vi "EyeTracking.vi"() -> ()   [LabVIEW 2010]
uses:
  <vilib>/vision/driver/IMAQdx.llb/IMAQdx Camera Control Mode.ctl
  <vilib>/vision/driver/NI_Vision_Acquisition_Software.lvlib
  Program Files/National Instruments/LabVIEW 2010/resource/objmgr/imaqdx.rc
  <vilib>/vision/driver/IMAQdx.llb/IMAQdx Acquisition Mode.ctl
  <vilib>/vision/NI_Vision_Development_Module.lvlib
  <vilib>/Utility/Variable/NI_VariableUtilities.lvlib
  <vilib>/DAQmx/write.llb/DAQmx Write (Analog 1D DBL NChan 1Samp).vi
  <vilib>/userDefined/High Color/IMAQdx.ctl
panel:
  out "IMAQ":bool
  out "acquired FPS":dbl
  out "processed FPS":dbl
  in  "Range":cluster{"Lower value":sgl, "Upper value":sgl}={"Lower value"=0.0, "Upper value"=29.0}
  in  "update FPS":u32=30
  out "Eye Trace":dbl[][](graph)
  in  "Pupil Color":sgl=150.0
  out "Centroid":cluster{"X Centroid":sgl, "Y Centroid":sgl} {"Y Centroid" format="%.2f"; "X Centroid" format="%.2f"}
  in  "Min Size":dbl=300.0
  in  "Max Size":dbl=25000.0
  in  "Despeckle":bool
  in  "desired FPS":dbl=200.0
  in  "AO Task":refnum<k21>="OpticalTrackerOut"
  in  "Track":bool
  out "Image":T1(plugin-control)
  in  "Session In":T2="cam0"
  in  "stop":bool
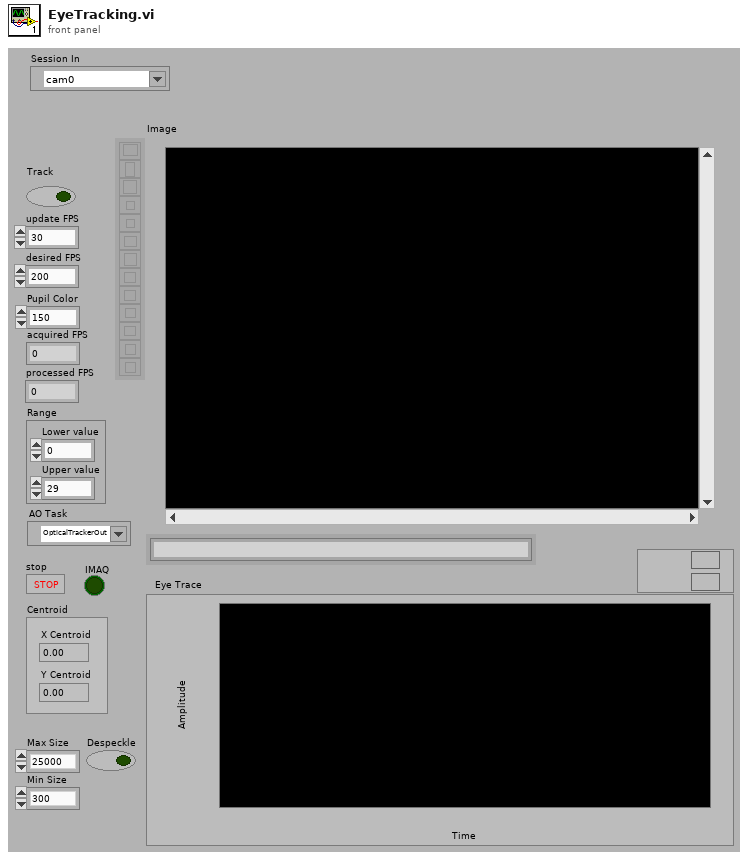
[diagram p1: front panel]
types:
  T1 = typedef "IMAQ Image.ctl" = refnum<image>
  T2 = typedef "IMAQdx.ctl" = refnum<k21>
  T3 = typedef "Image Type" = u32
  T4 = enum16{"Track", "Init Tracking", "Preview", "Init Preview"}
  T5 = cluster{"Type":u32, "Version":u32, "Flags":u32, "SerialNumberHigh":u32, "SerialNumberLow":u32, "BusType":u32, "InterfaceName":string, "VendorName":string, "ModelName":string, "CameraFileName":string, "CameraAttributeURL":string}[]
  T6 = typedef "NI_Vision_Acquisition_Software.lvlib/IMAQdx Camera Control Mode.ctl" = enum32{"Controller", "Listener"}
  T7 = typedef "NI_Vision_Acquisition_Software.lvlib/IMAQdx Acquisition Mode.ctl" = enum32{"One Shot", "Continuous"}
  T8 = cluster{"Global Rectangle":i32[], "Contours":cluster{"Contour Type":u32, "ROI Type":u32, "Points":i32[]}[]}
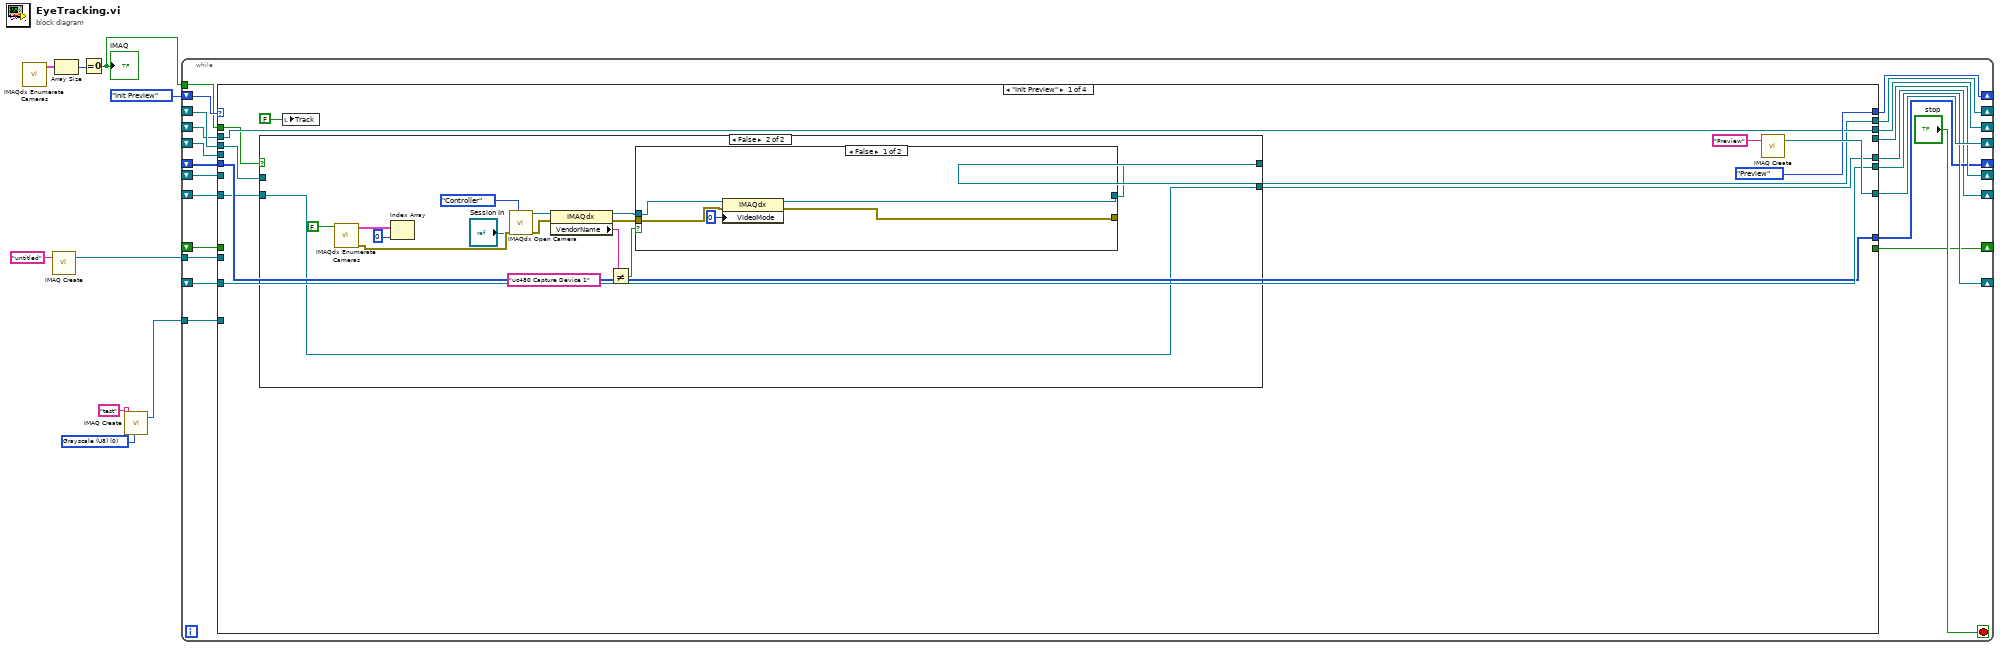
[diagram p0: block diagram]
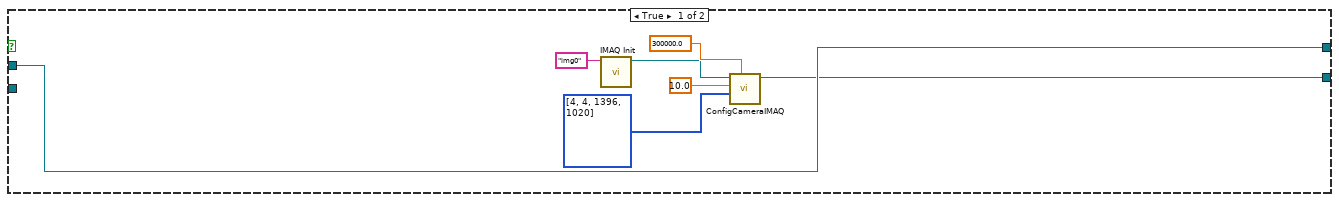
[diagram p2: hidden frame]
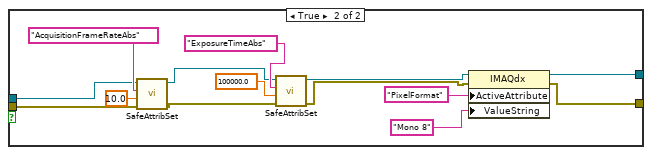
[diagram p3: hidden frame]
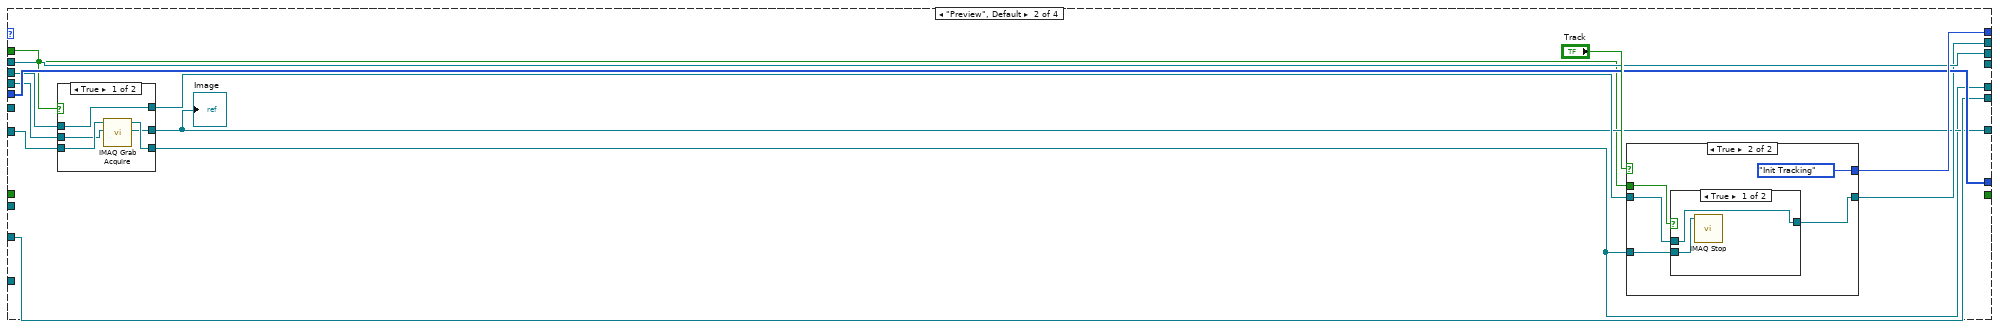
[diagram p4: hidden frame]
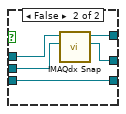
[diagram p5: hidden frame]
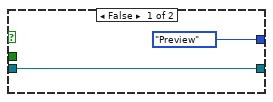
[diagram p6: hidden frame]
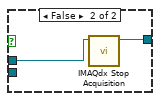
[diagram p7: hidden frame]
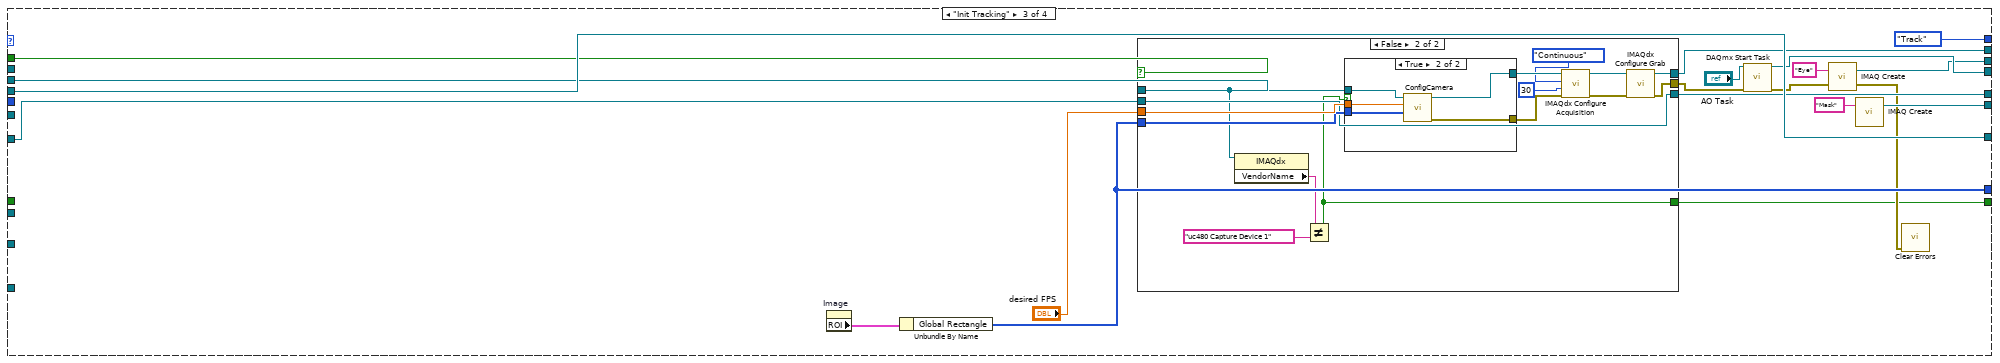
[diagram p8: hidden frame]
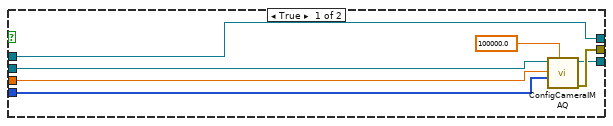
[diagram p9: hidden frame]
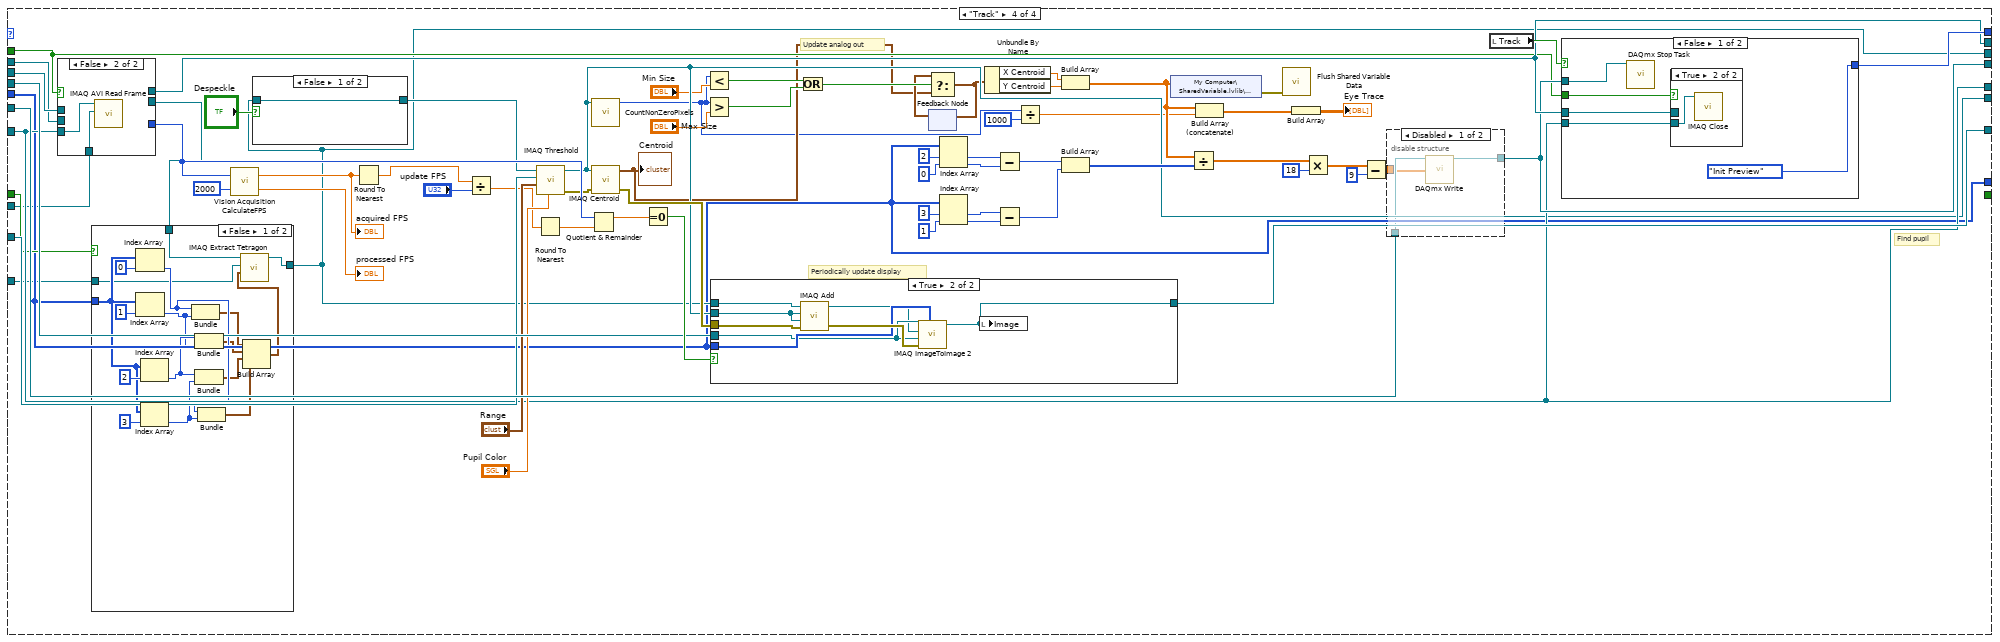
[diagram p11: hidden frame]
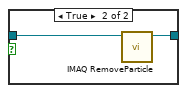
[diagram p14: hidden frame]
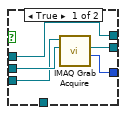
[diagram p15: hidden frame]
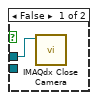
[diagram p17: hidden frame]
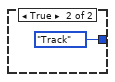
[diagram p18: hidden frame]
diagram:
  w5 = T3 0 items=["Grayscale (U8)", "Grayscale (I16)", "Grayscale (SGL)", "Complex (CSG)", "RGB (U32)", "HSL (U32)", "RGB (U64)", "Grayscale (U16)"] ("Image Type")
  n1 = call <vilib>:"IMAQdx Enumerate Cameras.vi"() -> ("Camera Information Array"=w8:T5)  [unwired: 2 in, 9 out]
  n2 = call "IMAQ Create"("Image Name"="untitled") -> ("New Image"=w1:T1)  [unwired: 4 in, 1 out]
  n3 = Array Size(array=w8) -> (size(s)=w7:i32)
  n4 = Equal To 0?(x=w7) -> (x = 0?=w6:bool)
  "IMAQ" <- w6
  n5 = call "IMAQ Create"("Image Name"="test", "Image Type"=w5) -> ("New Image"=w3:T1)  [unwired: 3 in, 1 out]
  n6 = while {
    shift-right: [w29] -> _
    shift-left: _ -> [w28]
    shift-right: [w27] -> _
    shift-left: _ -> [w26]
    shift-right: [w25] -> _
    shift-left: T4."Init Preview" -> [w30]
    shift-right: [w24] -> _
    shift-left: _ -> [w23]
    shift-right: [w22] -> _
    shift-left: _ -> [w21]
    shift-right: [w20] -> _
    shift-left: _ -> [w19]
    shift-right: [w18] -> _
    shift-left: _ -> [w17]
    tunnel: w6 -> [w16]
    shift-right: [w15] -> _
    shift-left: _ -> [w14]
    shift-right: [w13] -> _
    shift-left: _ -> [w12]
    tunnel: w3 -> [w11]
    tunnel: w1 -> [w10]
    stop <- "stop" stop-if-true
    n7 = case shown="\"Init Preview\"" w30 {
      tunnel: [w36 w88 w134 w229] -> w29
      tunnel: w28 -> [w34 w91 w123 w230]
      tunnel: [w42 w87 w136 w219] -> w27
      tunnel: w26 -> [_ w90 w136 w221]
      tunnel: [T4."Preview" w95 T4."Track" w232] -> w25
      tunnel: [_ _ w131 w225] -> w24
      tunnel: w23 -> [_ _ _ w228]
      tunnel: [w40 w94 w127 w169] -> w22
      tunnel: w21 -> [w40 w94 _ w220]
      tunnel: [w39 w92 w125 w188] -> w20
      tunnel: w19 -> [w39 w92 _ w202]
      tunnel: [w38 w93 w124 w168] -> w18
      tunnel: w17 -> [w38 w93 _ w168]
      tunnel: w16 -> [w35 w85 w122 w193]
      tunnel: [w33 w84 w120 w192] -> w15
      tunnel: w14 -> [w32 w86 w121 w192]
      tunnel: [_ _ w118 _] -> w13
      tunnel: w12 -> [_ _ _ w171]
      tunnel: w11 -> [_ _ _ w167]
      tunnel: w10 -> [_ _ _ w166]
      frame "Init Preview" {
        n8 = case shown="False" w35 {
          tunnel: [w50 w51] -> w36
          tunnel: w34 -> [w50 _]
          tunnel: [w46 w59] -> w33
          tunnel: w32 -> [_ w59]
          frame True {
            n9 = call <vilib>:"IMAQ Init.vi"("Interface Name"="img0") -> ("IMAQ Session Out"=w44:refnum<k11>)  [unwired: 1 in, 9 out]
            n10 = call "ConfigCameraIMAQ.vi"("desired exposure"=300000.0, "ROI"=i32[] [4, 4, 1396, 1020], "desired FPS"=10.0, "IMAQ Session In"=w44) -> ("IMAQ Session Out"=w46:refnum<k11>)  [unwired: 1 in, 6 out]
          }
          frame False {
            n11 = call <vilib>:"IMAQdx Enumerate Cameras.vi"("Connected Only? (Yes)"=FALSE) -> ("error out"=w61:errorcluster, "Camera Information Array"=w63:T5)  [unwired: 1 in, 8 out]
            n12 = Index Array(array=w63, index=0) -> ()  [unwired: 1 out]
            n13 = call <vilib>:"IMAQdx Open Camera.vi"("Camera Control Mode"=IMAQdx_Camera_Control_Mode."Controller", "error in"=w61, "Session In"="Session In") -> ("error out"=w56:errorcluster, "Session Out"=w57:T2)  [unwired: 7 out]
            n14 = property class="IMAQdx"(reference=w57, error in=w56) -> (error out=w55:errorcluster, "VendorName"=w54:string)  [unwired: 1 out]
            n15 = Not Equal?(x=w54, y="uc480 Capture Device 1") -> (x != y?=w53:bool)
            n16 = case shown="False" w53 {
              tunnel: [w67 w70] -> w51
              tunnel: [w66 w71] -> _
              tunnel: w57 -> [w69 w81]
              tunnel: w55 -> [w65 w80]
              frame False {
                n17 = property class="IMAQdx"(reference=w69, error in=w65, "VideoMode"=u32 0) -> (reference out=w67:T2, error out=w66:errorcluster)
              }
              frame True {
                n18 = call "SafeAttribSet.vi"("error in (no error)"=w80, "value"=10.0, "ActiveAttribute"="AcquisitionFrameRateAbs", "IMAQdx Session In"=w81) -> ("error out"=w76:errorcluster, "IMAQdx Session Out"=w77:T2)  [unwired: 6 out]
                n19 = call "SafeAttribSet.vi"("error in (no error)"=w76, "value"=100000.0, "ActiveAttribute"="ExposureTimeAbs", "IMAQdx Session In"=w77) -> ("error out"=w73:errorcluster, "IMAQdx Session Out"=w74:T2)  [unwired: 6 out]
                n20 = property class="IMAQdx"(reference=w74, error in=w73, "ActiveAttribute"="PixelFormat", "ValueString"="Mono 8") -> (reference out=w70:T2, error out=w71:errorcluster)
              }
            }
          }
        }
        n21 = local write "Track"(FALSE ("Track")) -> ()
        n22 = call "IMAQ Create"("Image Name"="Preview") -> ("New Image"=w42:T1)  [unwired: 3 in, 2 out]
      }
      frame "Preview", Default {
        n23 = case shown="True" w85 {
          tunnel: w91 -> [w101 w106]
          tunnel: [w98 w105] -> w87
          tunnel: w90 -> [w97 w104]
          tunnel: [w101 w103] -> w89
          tunnel: w86 -> [w100 w102]
          tunnel: [w99 w102] -> w84
          frame True {
            n24 = call <vilib>:"IMAQ Grab Acquire.vi"("Image In"=w97, "IMAQ Session In"=w100) -> ("Image Out"=w98:T1, "IMAQ Session Out"=w99:refnum<k11>)  [unwired: 3 in, 5 out]
          }
          frame False {
            n25 = call <vilib>:"IMAQdx Snap.vi"("Image In"=w104, "Session In"=w106) -> ("Image Out"=w105:T1, "Session Out"=w103:T2)  [unwired: 1 in, 7 out]
          }
        }
        "Image" <- w87
        n26 = case shown="True" "Track" {
          tunnel: [T4."Preview" T4."Init Tracking"] -> w95
          tunnel: w89 -> [w107 w112]
          tunnel: [w107 w111] -> w88
          tunnel: w85 -> [_ w110]
          tunnel: w84 -> [_ w109]
          frame False {
          }
          frame True {
            n27 = case shown="True" w110 {
              tunnel: w112 -> [w115 w117]
              tunnel: [w115 w116] -> w111
              tunnel: w109 -> [w114 _]
              frame True {
                n28 = call <vilib>:"IMAQ Stop.vi"("IMAQ Session In"=w114) -> ()  [unwired: 1 in, 10 out]
              }
              frame False {
                n29 = call <vilib>:"IMAQdx Stop Acquisition.vi"("Session In"=w117) -> ("Session Out"=w116:T2)  [unwired: 1 in, 9 out]
              }
            }
          }
        }
      }
      frame "Init Tracking" {
        n30 = property on="Image" class="ImageControl"() -> ("ROI"=w137:T8)  [unwired: 2 in, 2 out]
        n31 = Unbundle By Name(w137) -> ("Global Rectangle"=w124:i32[])
        n32 = case shown="False" w122 {
          tunnel: [w139 w159] -> w134
          tunnel: "desired FPS" -> [w143 w158]
          tunnel: [w141 w157] -> w130
          tunnel: w124 -> [w142 w156]
          tunnel: w123 -> [w139 w148]
          tunnel: w121 -> [w144 w151]
          tunnel: [w140 w151] -> w120
          tunnel: [_ w145] -> w118
          frame True {
            n33 = call "ConfigCameraIMAQ.vi"("desired exposure"=100000.0, "ROI"=w142, "desired FPS"=w143, "IMAQ Session In"=w144) -> ("error out"=w141:errorcluster, "IMAQ Session Out"=w140:refnum<k11>)  [unwired: 1 in, 5 out]
          }
          frame False {
            n34 = property class="IMAQdx"(reference=w148) -> ("VendorName"=w150:string)  [unwired: 1 in, 2 out]
            n35 = Not Equal?(x=w150, y="uc480 Capture Device 1") -> (x != y?=w145:bool)
            n36 = case shown="True" w145 {
              tunnel: w158 -> [_ w165]
              tunnel: w156 -> [_ w164]
              tunnel: [w160 w163] -> w155
              tunnel: [_ w162] -> w153
              tunnel: w148 -> [w160 w161]
              frame False {
              }
              frame True {
                n37 = call "ConfigCamera.vi"("ROI"=w164, "desired FPS"=w165, "Session In"=w161) -> ("error out"=w162:errorcluster, "IMAQdx Session Out"=w163:T2)  [unwired: 1 in, 6 out]
              }
            }
            n38 = call <vilib>:"IMAQdx Configure Acquisition.vi"("error in"=w153, "Number of Buffers"=u32 30, "Continuous?"=IMAQdx_Acquisition_Mode."Continuous", "Session In"=w155) -> ("error out"=w152:errorcluster, "Session Out"=w154:T2)  [unwired: 6 out]
            n39 = call <vilib>:"IMAQdx Configure Grab.vi"("error in"=w152, "Session In"=w154) -> ("error out"=w157:errorcluster, "Session Out"=w159:T2)  [unwired: 8 out]
          }
        }
        n40 = call <vilib>:"DAQmx Start Task.vi"("task/channels in"="AO Task", "error in"=w130) -> ("task out"=w131:refnum<k21>, "error out"=w128:errorcluster)  [unwired: 12 out]
        n41 = call "IMAQ Create"("Image Name"="Eye", "error in (no error)"=w128) -> ("New Image"=w127:T1, "error out"=w119:errorcluster)  [unwired: 2 in, 1 out]
        n42 = call "IMAQ Create"("Image Name"="Mask") -> ("New Image"=w125:T1)  [unwired: 3 in, 2 out]
        n43 = call <vilib>:"Clear Errors.vi"("error in (no error)"=w119) -> ()  [unwired: 6 in, 1 out]
      }
      frame "Track" {
        # "Periodically update display"
        # "Find pupil"
        # "Update analog out"
        n44 = case shown="False" w193 {
          tunnel: w230 -> [w262 _]
          tunnel: [w262 _] -> w229
          tunnel: [w259 _] -> w224
          tunnel: w220 -> [w261 _]
          tunnel: [w260 _] -> w170
          tunnel: w192 -> [w258 w263]
          tunnel: w166 -> [_ w264]
          frame True {
            n45 = call <vilib>:"IMAQ Grab Acquire.vi"("Image In"=w261, "IMAQ Session In"=w258) -> ("Acquired Buffer Number"=w259:u32, "Image Out"=w260:T1)  [unwired: 2 in, 6 out]
          }
          frame False {
            n46 = call "IMAQ AVI Read Frame"("Image"=w264, "Avi Refnum"=w263) -> ()  [unwired: 6 in, 4 out]
          }
        }
        n47 = case shown="False" w171 {
          tunnel: w170 -> [w248 w251]
          tunnel: [w247 w251] -> w169
          tunnel: w168 -> [w244 _]
          tunnel: w167 -> [w234 _]
          frame False {
            n48 = Index Array(array=w244, index=0) -> (element=w241:i32)
            n49 = Index Array(array=w244, index=1) -> (element=w242:i32)
            n50 = Index Array(array=w244, index=2) -> (element=w243:i32)
            n51 = Index Array(array=w244, index=3) -> (element=w240:i32)
            n52 = Bundle(w241, w242) -> (w239:cluster{i32, i32})  [unwired: 1 in]
            n53 = Bundle(w243, w242) -> (w238:cluster{i32, i32})  [unwired: 1 in]
            n54 = Bundle(w243, w240) -> (w237:cluster{i32, i32})  [unwired: 1 in]
            n55 = Bundle(w241, w240) -> (w236:cluster{i32, i32})  [unwired: 1 in]
            n56 = Build Array(w239, w238, w237, w236) -> (w235:cluster{i32, i32}[])
            n57 = call-poly "IMAQ Extract Tetragon"("Tetragon"=w235, "Image Dst"=w234, "Image Src"=w248) -> ("Image Dst Out"=w247:T1)  [unwired: 7 in, 1 out]
          }
          frame True {
          }
        }
        n58 = call <vilib>:"Vision Acquisition CalculateFPS.vi"("Update interval"=u32 2000, "buffer number"=w224) -> ("processed FPS"=→"processed FPS":dbl, "acquired FPS"=w191:dbl)
        "acquired FPS" <- w191
        n59 = case shown="False" "Despeckle" {
          tunnel: w169 -> [w255 w257]
          tunnel: [w255 w256] -> w173
          frame False {
          }
          frame True {
            n60 = call "IMAQ RemoveParticle"("Image Src"=w257) -> ("Image Dst Out"=w256:T1)  [unwired: 9 in, 1 out]
          }
        }
        n61 = Round To Nearest(number=w191) -> (nearest integer value=w190:dbl)
        n62 = Divide(x=w190, y="update FPS") -> (x/y=w196:dbl)
        n63 = Round To Nearest(number=w196) -> (nearest integer value=w195:dbl)
        n64 = call "IMAQ Threshold"("Replace Value"="Pupil Color", "Range"="Range", "Image Dst"=w202, "Image Src"=w173) -> ("error out"=w200:errorcluster, "Image Dst Out"=w188:T1)  [unwired: 2 in, 4 out]
        n65 = Quotient & Remainder(x=w224, y=w195) -> (x-y*floor(x/y)=w223:dbl)  [unwired: 1 out]
        n66 = call "CountNonZeroPixels.vi"("Image"=w188) -> ("NonZeroPixels"=w177:i32)  [unwired: 10 out]
        n67 = call "IMAQ Centroid"("error in (no error)"=w200, "Image"=w188) -> ("error out"=w198:errorcluster, "Centroid"=w179:cluster{"X Centroid":sgl, "Y Centroid":sgl})  [unwired: 1 in, 1 out]
        "Centroid" <- w179
        n68 = Equal To 0?(x=w223) -> (x = 0?=w222:bool)
        n69 = Less?(x=w177, y="Min Size") -> (x < y?=w183:bool)
        n70 = Greater?(x=w177, y="Max Size") -> (0:w182:bool)
        n71 = case shown="True" w222 {
          tunnel: w221 -> [w265 w268]
          tunnel: w169 -> [_ w273]
          tunnel: w188 -> [_ w272]
          tunnel: [w265 w269] -> w219
          tunnel: w168 -> [_ w270]
          tunnel: w198 -> [_ w267]
          frame False {
          }
          frame True {
            n72 = call "IMAQ Add"("Image Src A"=w273, "Image Dst"=w272, "Image Src B"=w272, "error in (no error)"=w267) -> ("Image Dst Out"=w266:T1, "error out"=w271:errorcluster)  [unwired: 1 in, 2 out]
            n73 = call "IMAQ ImageToImage 2"("Offset Left/Top"=w270, "error in (no error)"=w271, "Image Dst"=w268, "Image Src (Small)"=w266, "Image Src (Large)"=w268) -> ("Image Dst Out"=w269:T1)  [unwired: 1 in, 5 out]
            n74 = local write "Image"(w269) -> ()
          }
        }
        n75 = Or(x=w183, y=w182) -> (x .or. y?=w181:bool)
        n76 = feedback #1() -> (w180:cluster{"X Centroid":sgl, "Y Centroid":sgl})  [unwired: 1 out]
        n77 = Select(t=w180, s=w181, f=w179) -> (s? t:f=w178:cluster{"X Centroid":sgl, "Y Centroid":sgl})
        n78 = feedback-in #1(w178) -> ()
        n79 = Index Array(array=w168, index #1=2 ("index"), index #2=0 ("index")) -> (element #1=w213:i32, element #2=w214:i32)
        n80 = Index Array(array=w168, index #1=3 ("index"), index #2=1 ("index")) -> (element #1=w211:i32, element #2=w212:i32)
        n81 = Unbundle By Name(w178) -> ("X Centroid"=w227:sgl, "Y Centroid"=w226:sgl)
        n82 = Subtract(x=w213, y=w214) -> (x-y=w209:i32)
        n83 = Subtract(x=w211, y=w212) -> (x-y=w210:i32)
        n84 = Divide(x=w177, y=1000) -> (x/y=w175:dbl)
        n85 = Build Array(w227, w226) -> (w187:sgl[])
        n86 = Build Array(w209, w210) -> (w208:i32[])
        n87 = shared-variable "My Computer\\SharedVariable.lvlib\\EyePosition"(w187) -> (error out=w174:errorcluster)  [unwired: 1 out]
        n88 = Divide(x=w187, y=w208) -> (x/y=w207:sgl[])
        n89 = Build Array (concatenate)(w187, w175) -> (w186:dbl[])
        n90 = call <vilib>:"Flush Shared Variable Data.vi"("error in (no error)"=w174) -> ()  [unwired: 10 in, 1 out]
        n91 = Build Array(w186) -> (→"Eye Trace":dbl[][])
        n92 = Multiply(x=w207, y=18) -> (x*y=w205:sgl[])
        n93 = Subtract(x=w205, y=9) -> (x-y=w203:sgl[])
        n94 = disable-structure shown="Disabled" {
          disable-tunnel: w228 -> [w254 _]
          disable-tunnel: [w253 _] -> w225
          disable-tunnel: w203 -> [w252 _]
          frame Disabled {
            n95 = call-poly <vilib>:"DAQmx Write.vi"("task/channels in"=w254, "data"=w252) -> ("task out"=w253:refnum<k21>)  [unwired: 4 in, 9 out]
          }
          frame Enabled {
          }
        }
        n96 = local read "Track"() -> (w233:bool)
        n97 = case shown="False" w233 {
          tunnel: [T4."Init Preview" T4."Track"] -> w232
          tunnel: w229 -> [w277 _]
          tunnel: w225 -> [w276 _]
          tunnel: w193 -> [w275 _]
          tunnel: w192 -> [w274 _]
          frame False {
            n98 = call <vilib>:"DAQmx Stop Task.vi"("task/channels in"=w276) -> ()  [unwired: 1 in, 14 out]
            n99 = case shown="True" w275 {
              tunnel: w277 -> [w279 _]
              tunnel: w274 -> [_ w280]
              frame False {
                n100 = call <vilib>:"IMAQdx Close Camera.vi"("Session In"=w279) -> ()  [unwired: 1 in, 10 out]
              }
              frame True {
                n101 = call <vilib>:"IMAQ Close.vi"("IMAQ Session In"=w280) -> ()  [unwired: 1 in, 10 out]
              }
            }
          }
          frame True {
          }
        }
      }
    }
  }
